vi "Model.vi"(8 "error in (no error)":errorcluster) -> (0 "error out":errorcluster)   [LabVIEW 2021]
uses:
  QueueEnum.ctl
  ToViewQueueData.ctl
  ViewUpdateEnum.ctl
  ToControllerQueueCluster.ctl
  ToControllerEnum.ctl
  TCPQueueData.ctl
  TCPModuleState.ctl
panel:
  out "length":i32
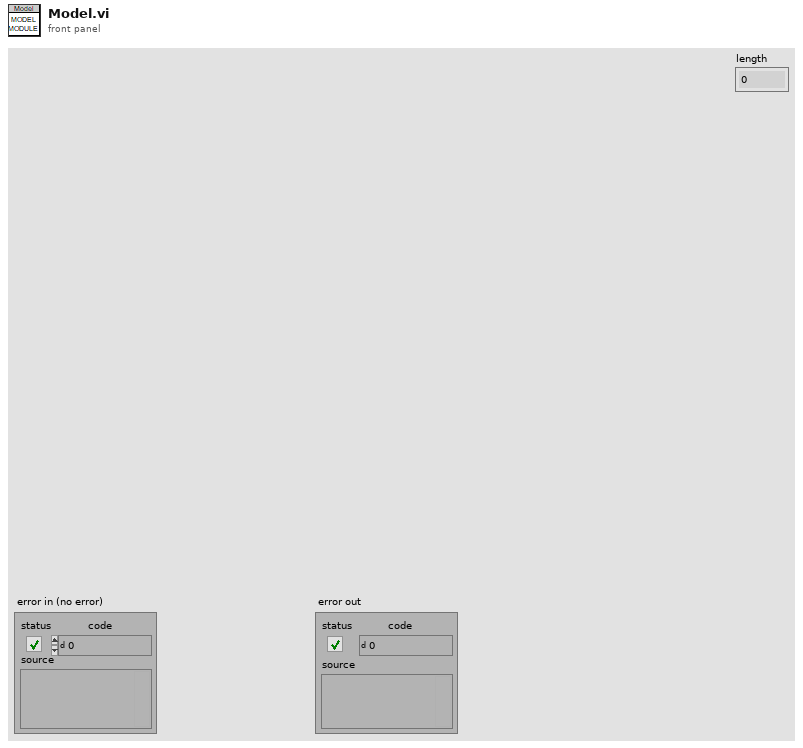
[diagram p1: front panel]
types:
  T1 = enum32{"Invalid", "Standard", "Closed", "Hidden", "Minimized", "Maximized"}
  T2 = typedef "QueueEnum.ctl" = enum16{"Obtain Queue", "Get Queue Ref", "Flush Queue", "Release Queue"}
  T3 = typedef "ViewUpdateEnum.ctl" = enum16{"OneButtonMessage", "Exit", "UpdateButtonsEnabled", "UpdateGraph", "UpdateConnectionStatus"}
  T4 = typedef "ToViewQueueData.ctl" = cluster{"DataToUpdate":T3, "ConnectionStatus":bool, "GraphData":dbl[][], "Message":string}
  T5 = typedef "ToControllerQueueCluster.ctl" = cluster{"Message":T6, "Remote IP":string, "Remote Port":u16, "Data":string}
  T6 = typedef "ToControllerEnum.ctl" = enum16{"Info_Disconnected", "Info_Connected", "Exit", "Disconnect", "Connect", "SendMessage"}
  T7 = typedef "TCPModuleState.ctl" = enum16{"Init", "Connect", "Read", "Write", "Disconnect", "ErrorHandler", "Exit"}
  T8 = typedef "TCPQueueData.ctl" = cluster{"Command":T7, "address":string, "remote port":u16, "Data":string}
  T9 = typedef "ModelQueueCluster.ctl" = cluster{"Source":T10, "FromTCPCluster":T11, "FromControllerCluster":T13}
  T10 = typedef "ToModelSourceEnum.ctl" = enum16{"TCP", "Controller"}
  T11 = typedef "FromTCPCluster.ctl" = cluster{"Message":T12, "Data":string, "StatusOK?":bool}
  T12 = typedef "ToModelFromTCPMessage.ctl" = enum16{"Exit", "DataWritten", "DataReceived", "Timeout", "UnableToConnect", "Disconnected", "Connected"}
  T13 = typedef "FormControllerToMOdelCluster.ctl" = cluster{"Command":T14, "IP Address":string, "Remote Port":u16, "Data":string}
  T14 = typedef "ToModelFromControllerEnum.ctl" = enum16{"SendMessage", "Exit", "Disconnect", "Connect"}
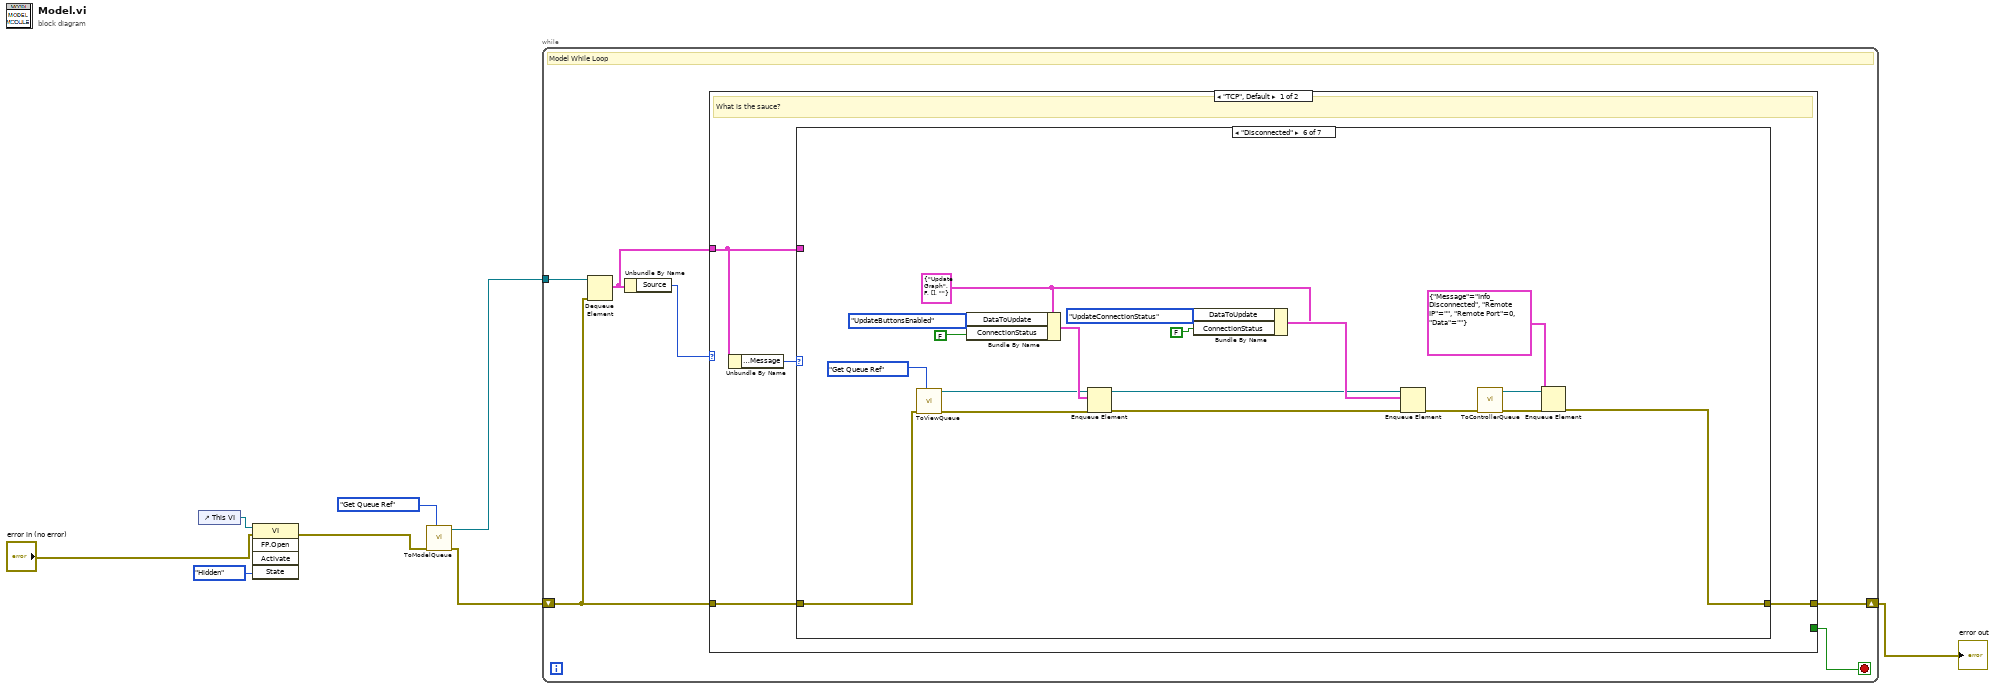
[diagram p0: block diagram]
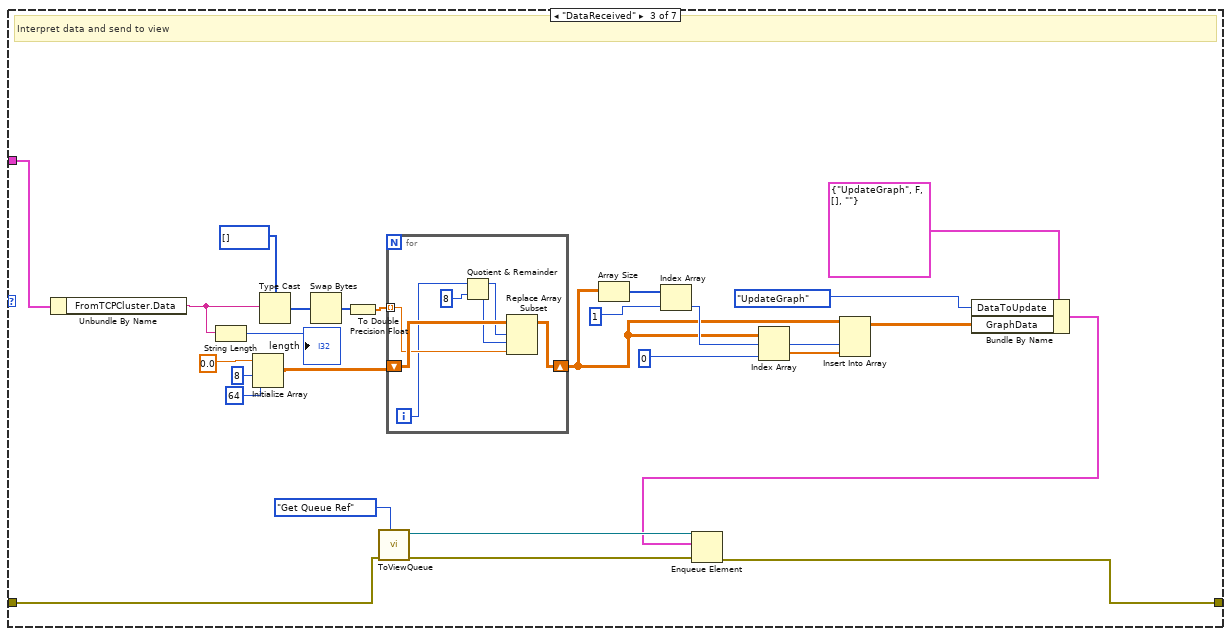
[diagram p4: hidden frame]
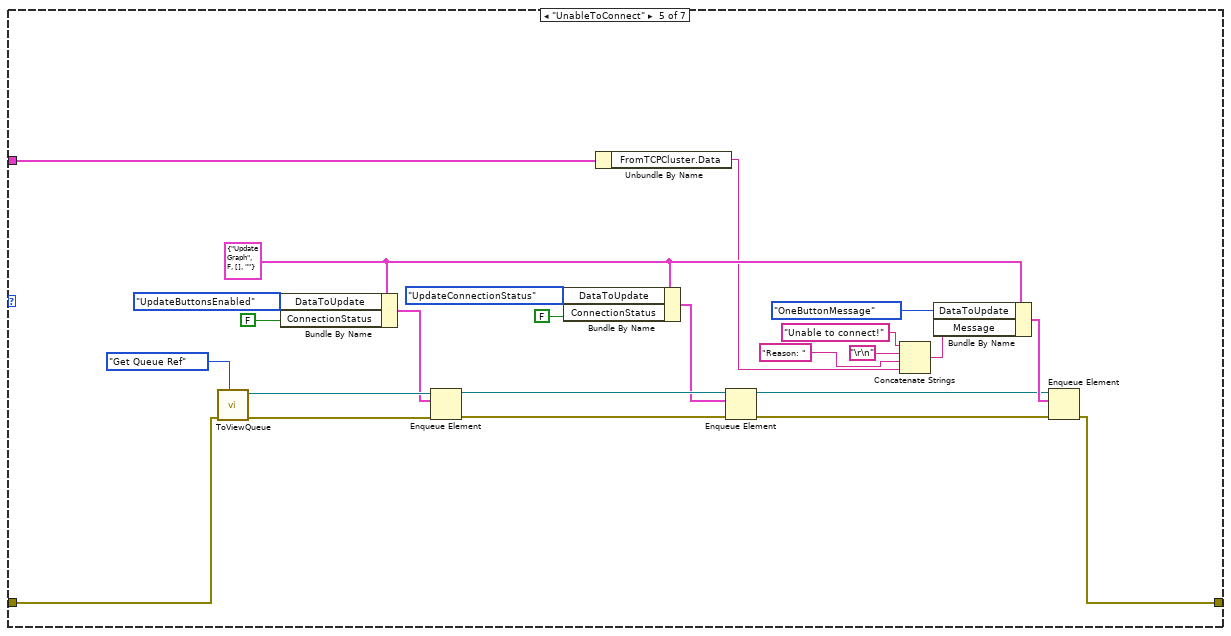
[diagram p6: hidden frame]
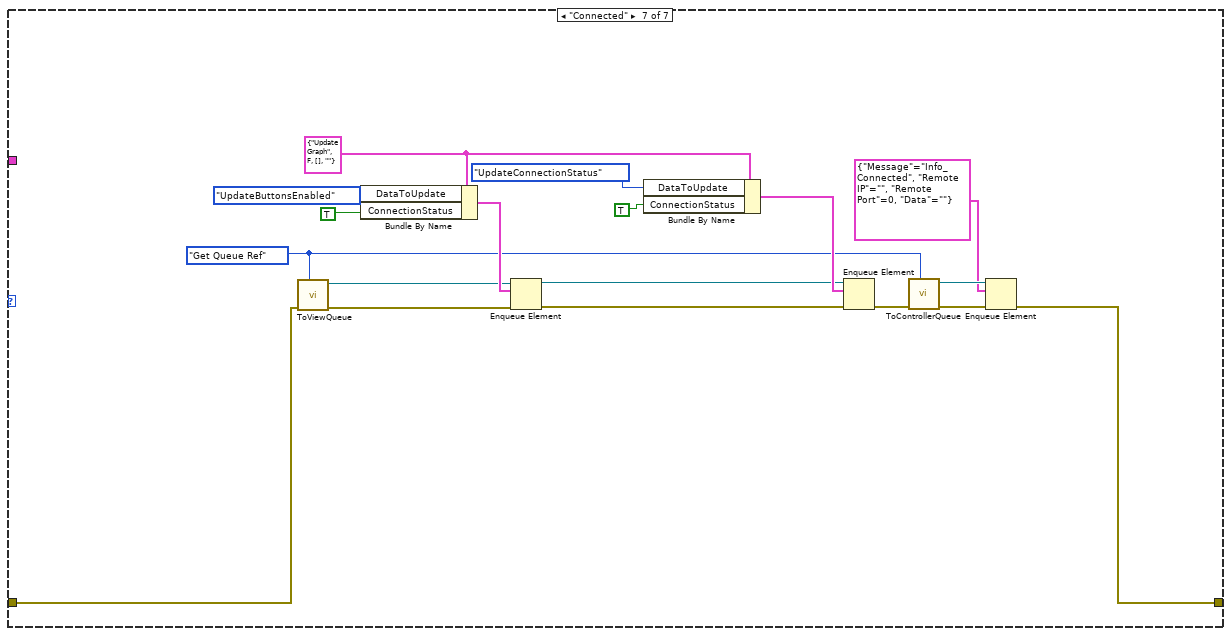
[diagram p7: hidden frame]
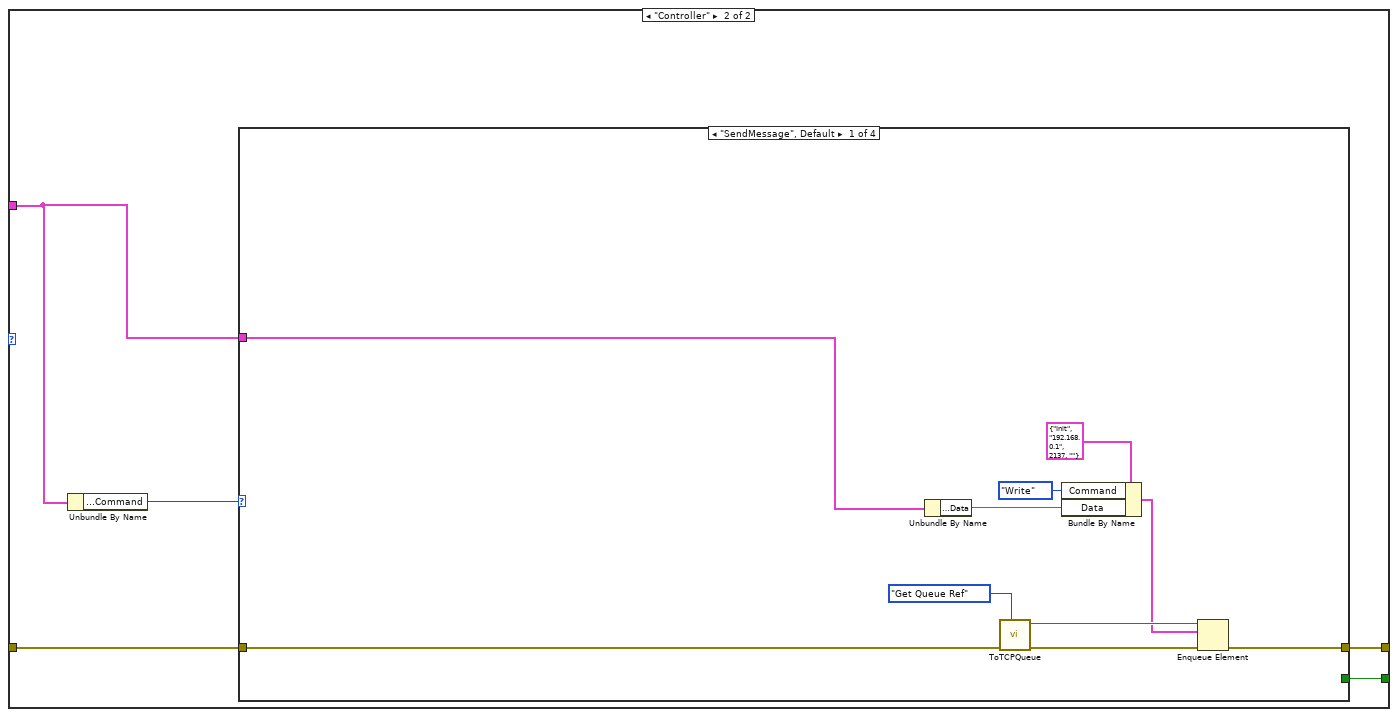
[diagram p8: hidden frame]
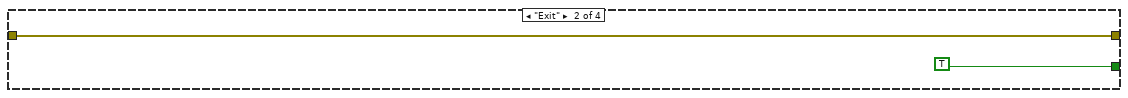
[diagram p9: hidden frame]
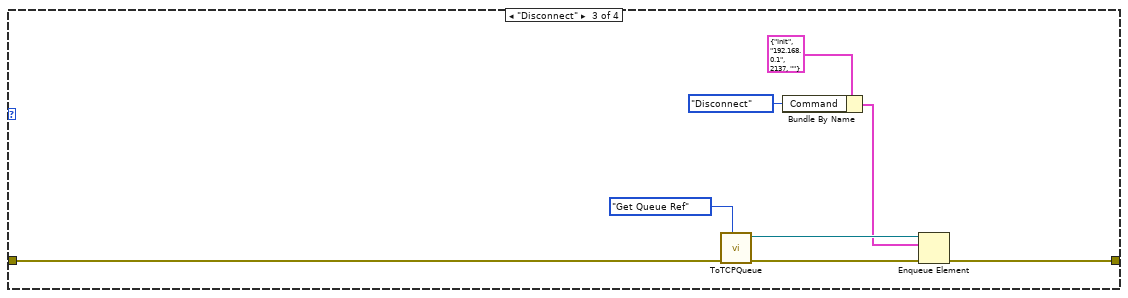
[diagram p10: hidden frame]
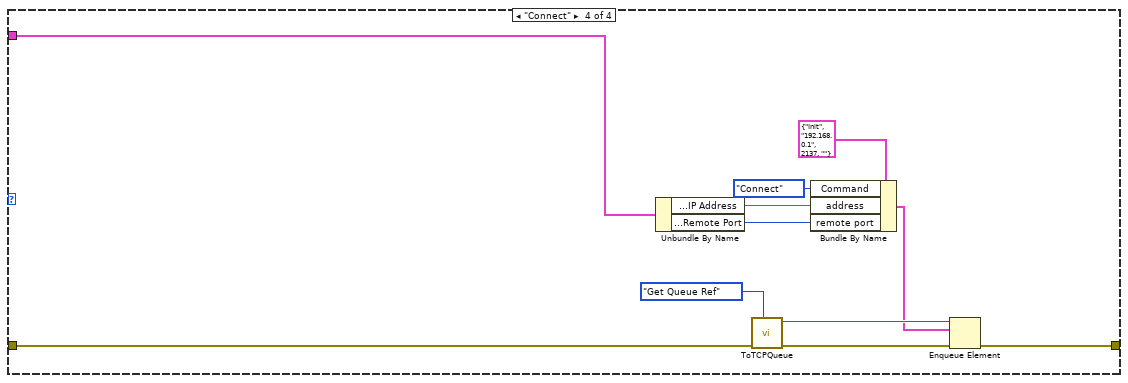
[diagram p11: hidden frame]
diagram:
  n1 = control-ref of="This VI"() -> (w4:refnum<vi>)
  n2 = invoke class="VI" method="FP.Open"(reference=w4, error in="error in (no error)", "State"=T1."Hidden") -> (error out=w1:errorcluster)  [unwired: 2 in, 4 out]
  n3 = call "ToModelQueue.vi"("Enum"=QueueEnum."Get Queue Ref", "error in (no error)"=w1) -> ("error out"=w8:errorcluster, "queue out"=w6:refnum<queue>)  [unwired: 8 in]
  n4 = while {
    tunnel: w6 -> [w14]
    shift-right: [w9] -> w5
    shift-left: w8 -> [w10]
    stop <- w11 stop-if-true
    # "Model While Loop"
    n5 = Dequeue Element(queue=w14, error in (no error)=w10) -> (element=w12:T9)  [unwired: 1 in, 3 out]
    n6 = Unbundle By Name(w12) -> ("Source"=w13:T10)
    n7 = case shown="\"TCP\", Default" w13 {
      tunnel: w12 -> [w15 w117]
      tunnel: [_ w118] -> w11
      tunnel: w10 -> [w17 w116]
      tunnel: [w16 w115] -> w9
      frame "TCP", Default {
        # "What is the sauce?"
        n8 = Unbundle By Name(w15) -> ("FromTCPCluster.Message"=w18:T12)
        n9 = case shown="\"Disconnected\"" w18 {
          tunnel: w17 -> [w19 w20 w23 w54 w78 w84 w103]
          tunnel: [w19 w20 w22 w54 w66 w81 w100] -> w16
          tunnel: w15 -> [_ _ w31 _ w60 _ _]
          frame "Exit", Default {
            # "Nothing to do"
          }
          frame "DataWritten" {
            # "Thats good! Nothing to do"
          }
          frame "DataReceived" {
            # "Interpret data and send to view"
            n10 = Unbundle By Name(w31) -> ("FromTCPCluster.Data"=w30:string)
            n11 = String Length(string=w30) -> (length=→"length":i32)
            n12 = Initialize Array(0.0 ("element"), 8 ("dimension size"), 64 ("dimension size")) -> (w40:dbl[][])
            n13 = Type Cast(type=u16[] [], x=w30) -> (*(type *) &x=w45:u16[])
            n14 = Swap Bytes(anything=w45) -> (byte swapped=w38:u16[])
            n15 = To Double Precision Float(number=w38) -> (double precision float=w44:dbl[])
            n16 = call "ToViewQueue.vi"("Enum"=QueueEnum."Get Queue Ref", "error in (no error)"=w23) -> ("error out"=w29:errorcluster, "queue out"=w28:refnum<queue>)  [unwired: 8 in]
            n17 = for {
              tunnel: w44 -> [w49] mode=indexing
              shift-right: [w51] -> w34
              shift-left: w40 -> [w53]
              i -> [w47]
              n18 = Quotient & Remainder(x=w47, y=8 ("x")) -> (x-y*floor(x/y)=w52:i32, floor(x/y)=w50:i32)
              n19 = Replace Array Subset(array=w53, new element=w49, index (row)=w52, index (col)=w50) -> (w51:dbl[][])
            }
            n20 = Array Size(array=w34) -> (size(s)=w37:i32[])
            n21 = Index Array(array=w37, index=1) -> (element=w35:i32)
            n22 = Index Array(array=w34, index (col)=0 ("disabled index (col)")) -> (element=w32:dbl[])  [unwired: 1 in]
            n23 = Insert Into Array(array=w34, index (col)=w35, new element=w32) -> (w26:dbl[][])  [unwired: 1 in]
            n24 = Bundle By Name(cluster=T4 {"DataToUpdate"=enum."UpdateGraph", "ConnectionStatus"=FALSE, "GraphData"=[], "Message"=""} ("element"), "DataToUpdate"=ViewUpdateEnum."UpdateGraph", "GraphData"=w26) -> (w24:T4)
            n25 = Enqueue Element(queue=w28, element=w24, error in (no error)=w29) -> (error out=w22:errorcluster)  [unwired: 1 in, 2 out]
          }
          frame "Timeout" {
            # "Nothing to do"
          }
          frame "UnableToConnect" {
            w64 = T4 {"DataToUpdate"=enum."UpdateGraph", "ConnectionStatus"=FALSE, "GraphData"=[], "Message"=""} ("element")
            n26 = call "ToViewQueue.vi"("Enum"=QueueEnum."Get Queue Ref", "error in (no error)"=w78) -> ("error out"=w76:errorcluster, "queue out"=w75:refnum<queue>)  [unwired: 8 in]
            n27 = Bundle By Name(cluster=w64, "DataToUpdate"=ViewUpdateEnum."UpdateButtonsEnabled", "ConnectionStatus"=FALSE) -> (w73:T4)
            n28 = Enqueue Element(queue=w75, element=w73, error in (no error)=w76) -> (queue out=w70:refnum<queue>, error out=w71:errorcluster)  [unwired: 1 in, 1 out]
            n29 = Bundle By Name(cluster=w64, "DataToUpdate"=ViewUpdateEnum."UpdateConnectionStatus", "ConnectionStatus"=FALSE) -> (w68:T4)
            n30 = Unbundle By Name(w60) -> ("FromTCPCluster.Data"=w56:string)
            n31 = Enqueue Element(queue=w70, element=w68, error in (no error)=w71) -> (queue out=w61:refnum<queue>, error out=w65:errorcluster)  [unwired: 1 in, 1 out]
            n32 = Concatenate Strings("Unable to connect!" ("Message"), "\r\n", "Reason: " ("string"), w56) -> (w59:string)
            n33 = Bundle By Name(cluster=w64, "DataToUpdate"=ViewUpdateEnum."OneButtonMessage", "Message"=w59) -> (w62:T4)
            n34 = Enqueue Element(queue=w61, element=w62, error in (no error)=w65) -> (error out=w66:errorcluster)  [unwired: 1 in, 2 out]
          }
          frame "Disconnected" {
            w89 = T4 {"DataToUpdate"=enum."UpdateGraph", "ConnectionStatus"=FALSE, "GraphData"=[], "Message"=""} ("element")
            n35 = call "ToViewQueue.vi"("Enum"=QueueEnum."Get Queue Ref", "error in (no error)"=w84) -> ("error out"=w91:errorcluster, "queue out"=w92:refnum<queue>)  [unwired: 8 in]
            n36 = Bundle By Name(cluster=w89, "DataToUpdate"=ViewUpdateEnum."UpdateButtonsEnabled", "ConnectionStatus"=FALSE) -> (w93:T4)
            n37 = Enqueue Element(queue=w92, element=w93, error in (no error)=w91) -> (queue out=w95:refnum<queue>, error out=w94:errorcluster)  [unwired: 1 in, 1 out]
            n38 = Bundle By Name(cluster=w89, "DataToUpdate"=ViewUpdateEnum."UpdateConnectionStatus", "ConnectionStatus"=FALSE) -> (w96:T4)
            n39 = Enqueue Element(queue=w95, element=w96, error in (no error)=w94) -> (error out=w83:errorcluster)  [unwired: 1 in, 2 out]
            n40 = call "ToControllerQueue.vi"("error in (no error)"=w83) -> ("error out"=w82:errorcluster, "queue out"=w80:refnum<queue>)  [unwired: 9 in]
            n41 = Enqueue Element(queue=w80, element=T5 {"Message"=enum."Info_Disconnected", "Remote IP"="", "Remote Port"=0, "Data"=""}, error in (no error)=w82) -> (error out=w81:errorcluster)  [unwired: 1 in, 2 out]
          }
          frame "Connected" {
            w108 = T4 {"DataToUpdate"=enum."UpdateGraph", "ConnectionStatus"=FALSE, "GraphData"=[], "Message"=""} ("element")
            w98 = QueueEnum."Get Queue Ref"
            n42 = call "ToViewQueue.vi"("Enum"=w98, "error in (no error)"=w103) -> ("error out"=w109:errorcluster, "queue out"=w110:refnum<queue>)  [unwired: 8 in]
            n43 = Bundle By Name(cluster=w108, "DataToUpdate"=ViewUpdateEnum."UpdateButtonsEnabled", "ConnectionStatus"=TRUE) -> (w111:T4)
            n44 = Enqueue Element(queue=w110, element=w111, error in (no error)=w109) -> (queue out=w113:refnum<queue>, error out=w112:errorcluster)  [unwired: 1 in, 1 out]
            n45 = Bundle By Name(cluster=w108, "DataToUpdate"=ViewUpdateEnum."UpdateConnectionStatus", "ConnectionStatus"=TRUE) -> (w114:T4)
            n46 = Enqueue Element(queue=w113, element=w114, error in (no error)=w112) -> (error out=w102:errorcluster)  [unwired: 1 in, 2 out]
            n47 = call "ToControllerQueue.vi"("Enum"=w98, "error in (no error)"=w102) -> ("error out"=w101:errorcluster, "queue out"=w99:refnum<queue>)  [unwired: 8 in]
            n48 = Enqueue Element(queue=w99, element=T5 {"Message"=enum."Info_Connected", "Remote IP"="", "Remote Port"=0, "Data"=""}, error in (no error)=w101) -> (error out=w100:errorcluster)  [unwired: 1 in, 2 out]
          }
        }
      }
      frame "Controller" {
        n49 = Unbundle By Name(w117) -> ("FromControllerCluster.Command"=w119:T14)
        n50 = case shown="\"SendMessage\", Default" w119 {
          tunnel: [_ TRUE _ _] -> w118
          tunnel: w117 -> [w120 _ _ w140]
          tunnel: w116 -> [w122 w130 w138 w142]
          tunnel: [w121 w130 w132 w141] -> w115
          frame "SendMessage", Default {
            n51 = Unbundle By Name(w120) -> ("FromControllerCluster.Data"=w124:string)
            n52 = call "ToTCPQueue.vi"("Enum"=QueueEnum."Get Queue Ref", "error in (no error)"=w122) -> ("error out"=w128:errorcluster, "queue out"=w127:refnum<queue>)  [unwired: 8 in]
            n53 = Bundle By Name(cluster=T8 {"Command"=enum."Init", "address"="192.168.0.1", "remote port"=2137, "Data"=""} ("element"), "Command"=TCPModuleState."Write", "Data"=w124) -> (w123:T8)
            n54 = Enqueue Element(queue=w127, element=w123, error in (no error)=w128) -> (error out=w121:errorcluster)  [unwired: 1 in, 2 out]
          }
          frame "Exit" {
          }
          frame "Disconnect" {
            n55 = call "ToTCPQueue.vi"("Enum"=QueueEnum."Get Queue Ref", "error in (no error)"=w138) -> ("error out"=w137:errorcluster, "queue out"=w136:refnum<queue>)  [unwired: 8 in]
            n56 = Bundle By Name(cluster=T8 {"Command"=enum."Init", "address"="192.168.0.1", "remote port"=2137, "Data"=""} ("element"), "Command"=TCPModuleState."Disconnect") -> (w133:T8)
            n57 = Enqueue Element(queue=w136, element=w133, error in (no error)=w137) -> (error out=w132:errorcluster)  [unwired: 1 in, 2 out]
          }
          frame "Connect" {
            n58 = Unbundle By Name(w140) -> ("FromControllerCluster.IP Address"=w145:string, "FromControllerCluster.Remote Port"=w144:u16)
            n59 = call "ToTCPQueue.vi"("Enum"=QueueEnum."Get Queue Ref", "error in (no error)"=w142) -> ("error out"=w149:errorcluster, "queue out"=w148:refnum<queue>)  [unwired: 8 in]
            n60 = Bundle By Name(cluster=T8 {"Command"=enum."Init", "address"="192.168.0.1", "remote port"=2137, "Data"=""} ("element"), "Command"=TCPModuleState."Connect", "address"=w145, "remote port"=w144) -> (w143:T8)
            n61 = Enqueue Element(queue=w148, element=w143, error in (no error)=w149) -> (error out=w141:errorcluster)  [unwired: 1 in, 2 out]
          }
        }
      }
    }
  }
  "error out" <- w5
